vi "Lockin Engine.vi"(8 "error in (no error)":errorcluster, 9 "REF Waveforms":waveform(dbl)[](array[waveform]), 10 "AI Waveforms":waveform(dbl)[](array[waveform]), 11 "LockinDAQ":refnum<class "LockinDAQ.lvclass">) -> (0 "error out":errorcluster, 1 "SweepResults":T1, 2 "Averaged Results (X,Y,R,Theta,Mean)":T2 {"Results" format="%#_6p"}, 3 "LockinDAQ out":refnum<class "LockinDAQ.lvclass">)   [LabVIEW 2016, in "LockinDAQ.lvclass"]
uses:
  LockinDAQ.lvclass
  Typedefs/Results--Cluster.ctl
  Typedefs/SweepResults--Cluster.ctl
  LockinDAQ.lvclass/LockinDAQ.ctl
  <vilib>/Analysis/baseanly.llb/Mean (DBL).vi
  <vilib>/ptbypt/Filters.llb/Butterworth Filter PtByPt.vi
  <vilib>/Analysis/3filter.llb/Butterworth Filter.vi
  <vilib>/Analysis/3filter.llb/Butterworth Filter (DBL).vi
  <vilib>/addons/System Identification/Data Preprocess.llb/SI Lowpass Filter.vi
  <vilib>/addons/System Identification/Data Preprocess.llb/SI Lowpass Filter (SISO Waveform).vi
  <vilib>/addons/Digital Filter Design/Process.llb/DFD Filtering (Wfm NChan).vi
  <vilib>/measure/maresamp.llb/Resample Waveforms (single shot).vi
  <vilib>/measure/maresamp.llb/Resample Waveform (single shot).vi
  <vilib>/Analysis/NI_AALBase.lvlib
  <vilib>/addons/Digital Filter Design/NI_DigFilterLicensed.lvlib
panel:
  out "Results (Ch1)":cluster{i32[], dbl[]}[](graph)
  out "filter fC (Hz)":dbl=0.3183098861837907
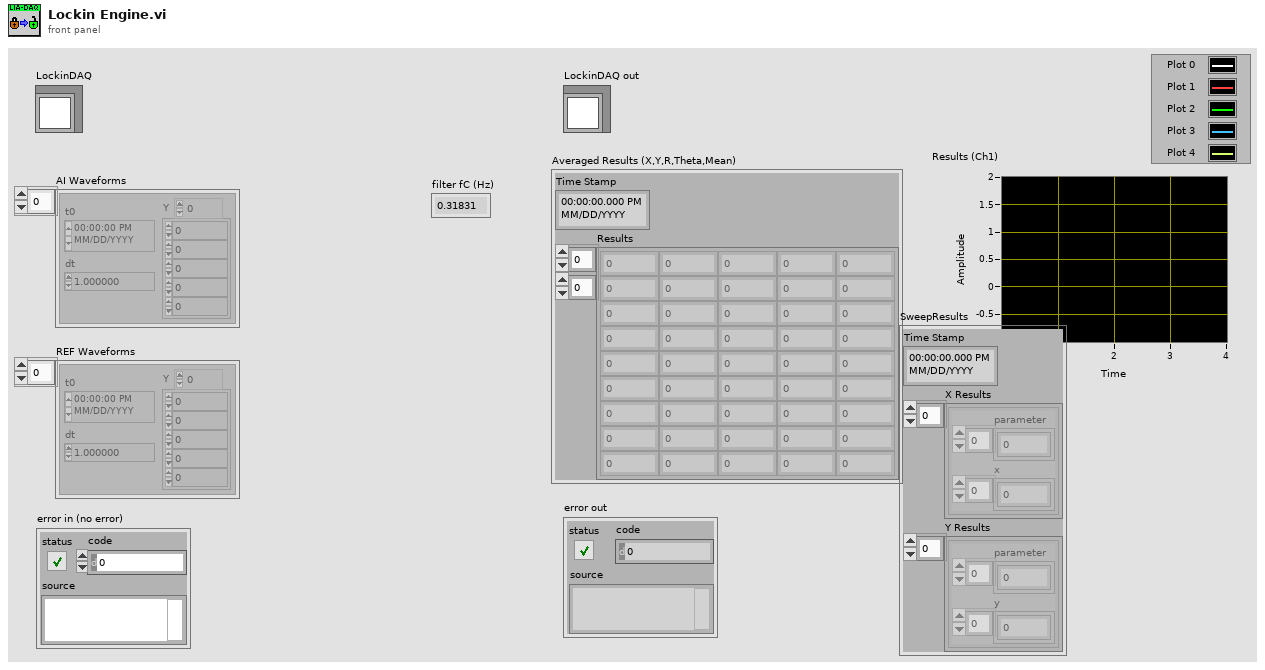
[diagram p1: front panel]
types:
  T1 = typedef "LockinDAQ.lvclass/SweepResults--Cluster.ctl" = cluster{"Time Stamp":timestamp, "X Results":cluster{"parameter":dbl[], "x":dbl[]}[], "Y Results":cluster{"parameter":dbl[], "y":dbl[]}[]}
  T2 = typedef "LockinDAQ.lvclass/Results--Cluster.ctl" = cluster{"Time Stamp":timestamp, "Results":dbl[][]}
  T3 = enum16{"method 1", "method 2", "method 3", "method 4", "method 5"}
  T4 = enum16{"Lowpass", "Highpass", "Bandpass", "Bandstop"}
  T5 = typedef "NI_DigFilterLicensed.lvlib/DFD Filter Obj.ctl" = cluster{"mSRate_Fs":dbl, "mSRate_Version":string, "mSRate_Comments":string, "mSRate_OrgCoef":T6, "mSRate_CurCoef":T6, "mSRate_Quantized?":bool, "mSRate_QCoef":T6, "mSRate_QSettings":T8[], "mSRate_Order":i32, "mSRate_Scaling":cluster{"mSRate_ScaleByPowerOf2?":bool, "mSRate_ScaleType":T10}}
  T6 = typedef "NI_DigFilterLicensed.lvlib/DFD Filter Coef.ctl" = cluster{"type":T7, "gain":dbl, "coef a (k)":dbl[], "coef b (v)":dbl[]}
  T7 = typedef "NI_DigFilterLicensed.lvlib/DFD Filter Structure Type Selector.ctl" = enum16{"Undefined", "FIR Direct Form", "FIR Direct Form Transposed", "FIR Symmetric", "FIR Antisymmetric", "IIR Direct Form I", "IIR Direct Form I Transposed", "IIR Direct Form II", "IIR Direct Form II Transposed", "IIR Cascaded Second Order Sections Form I", "IIR Cascaded Second Order Sections Form I Transposed", "IIR Cascaded Second Order Sections Form II", "IIR Cascaded Second Order Sections Form II Transposed", "Lattice Allpass (basic sections)", "Lattice Allpass (one multiplier sections)", "Lattice Allpass (normalized sections)", "Lattice AR (basic sections)", "Lattice AR (one multiplier sections)", "Lattice AR (normalized sections)", "Lattice MA (minimum phase)", "Lattice MA (maximum phase)", "Lattice ARMA (basic sections)", "Lattice ARMA (one multiplier sections)", "Lattice ARMA (normalized sections)"}
  T8 = typedef "NI_DigFilterLicensed.lvlib/dfd_Internal Quantization Settings.ctl" = cluster{"source":T9, "wl":i16, "iwl":i16, "overflow mode":enum16{"Saturation", "Wrap"}, "rounding mode":enum16{"Nearest", "Truncation"}, "signed?":bool}
  T9 = typedef "NI_DigFilterLicensed.lvlib/dfd_Internal Quantization Srcs.ctl" = u16
  T10 = typedef "NI_DigFilterLicensed.lvlib/DFD Coef Norm Type.ctl" = enum16{"No Norm", "Time Domain 1-Norm", "Time Domain 2-Norm", "Time Domain Inf-Norm"}
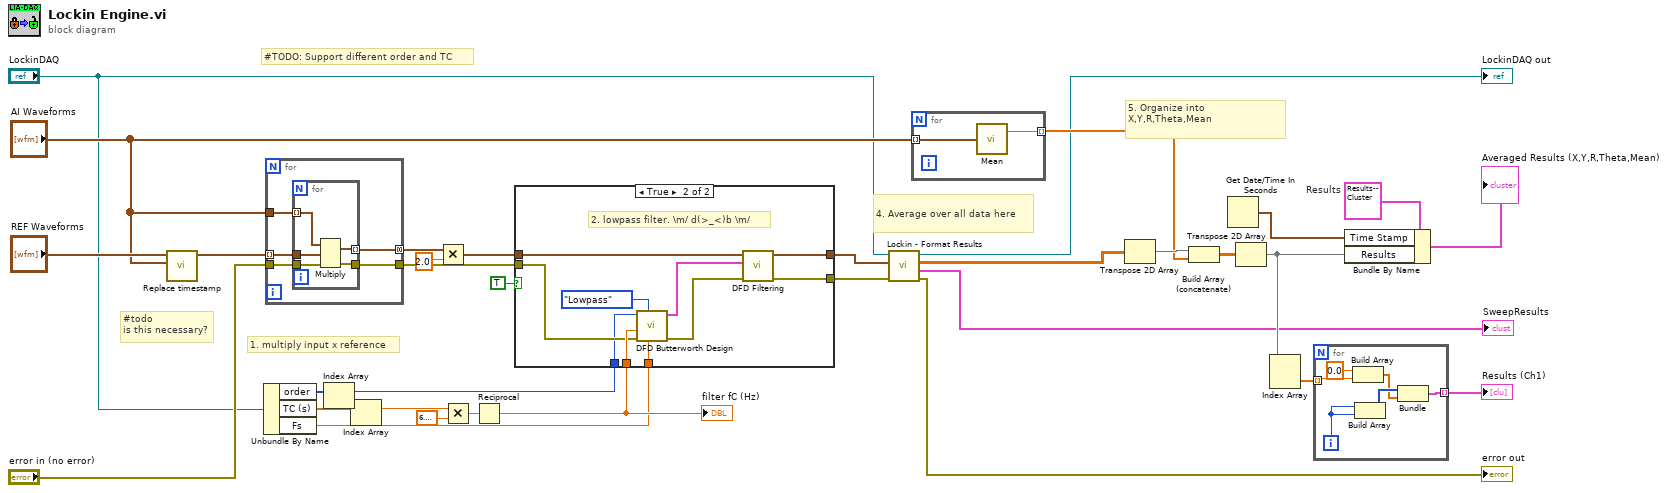
[diagram p0: block diagram]
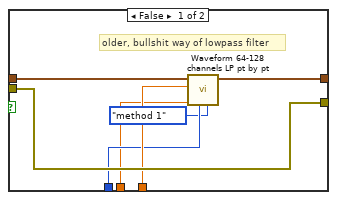
[diagram p2: hidden frame]
diagram:
  w27 = T2 {"Time Stamp"=timestamp(0 s since 1904-01-01), "Results"=[]}  # Results
  # "#TODO: Support different order and TC"
  # "#todo\nis this necessary?"
  # "5. Organize into X,Y,R,Theta,Mean"
  # "4. Average over all data here"
  # "1. multiply input x reference"
  n1 = call "Replace timestamp.vi"("Array in (use this time stamp)"="AI Waveforms", "Array in"="REF Waveforms") -> ("Array out"=w33:waveform(dbl)[])  [unwired: 9 in]
  n2 = Unbundle By Name("LockinDAQ") -> ("order"=w15:i32[], "TC (s)"=w30:dbl[], "Fs"=w16:dbl)
  n3 = for {
    tunnel: [w38] -> w24 mode=concatenating
    tunnel: w33 -> [w37] mode=indexing
    tunnel: "AI Waveforms" -> [w36]
    tunnel: [w35] -> w17
    tunnel: "error in (no error)" -> [w34]
    n4 = for {
      tunnel: w36 -> [w42] mode=indexing
      tunnel: w37 -> [w41]
      tunnel: [w43] -> w38 mode=indexing
      tunnel: [w40] -> w35
      tunnel: w34 -> [w39]
      n5 = Multiply(1:w41, 2:w42, 4:w39) -> (0:w43:waveform(dbl), 3:w40:errorcluster)
    }
  }
  n6 = Index Array(array=w15) -> (element=w2:i32)  [unwired: 1 in]
  n7 = Index Array(array=w30) -> (element=w1:dbl)  [unwired: 1 in]
  n8 = Multiply(x=w24, y=2.0) -> (x*y=w19:waveform(dbl)[])
  n9 = Multiply(x=w1, y=6.283185307179586) -> (x*y=w32:dbl)
  n10 = Reciprocal(x=w32) -> (1/x=w18:dbl)
  "filter fC (Hz)" <- w18
  n11 = case shown="True" TRUE {
    tunnel: w19 -> [w50 w58]
    tunnel: [w49 w57] -> w6
    tunnel: w18 -> [w45 w56]
    tunnel: w17 -> [w48 w55]
    tunnel: w16 -> [w47 w54]
    tunnel: w2 -> [w46 w53]
    tunnel: [w48 w51] -> w9
    frame False {
      # "older, bullshit way of lowpass filter"
      n12 = call "Waveform 64-128 channels LP pt by pt.vi"("Enum"=T3."method 1", "order"=w46, "fl"=w45, "fs"=w47, "Array in"=w50) -> ("Array out"=w49:waveform(dbl)[])  [unwired: 6 in]
    }
    frame True {
      # "2. lowpass filter. \\m/ d(>_<)b \\m/"
      n13 = call <vilib>:"DFD Butterworth Design.vi"("fs [Hz]"=w54, "filter type"=T4."Lowpass", "error in (no error)"=w55, "low cutoff freq [Hz]"=w56, "order"=w53) -> ("error out"=w59:errorcluster, "filter out"=w60:T5)  [unwired: 5 in]
      n14 = call-poly <vilib>:"DFD Filtering.vi"("error in (no error)"=w59, "filter"=w60, "signal in"=w58) -> ("error out"=w51:errorcluster, "signal out"=w57:waveform(dbl)[])  [unwired: 7 in]
    }
  }
  n15 = call "Lockin - Format Results.vi"("error in (no error)"=w9, "signal in"=w6, "LockinDAQ"="LockinDAQ") -> ("error out"=→"error out":errorcluster, "SweepResults"=→"SweepResults":T1, "Results (X,Y,R,Theta)"=w3:dbl[][], "LockinDAQ out"=→"LockinDAQ out":refnum<class "LockinDAQ.lvclass">)  [unwired: 5 in]
  n16 = for {
    tunnel: "AI Waveforms" -> [w62] mode=indexing
    tunnel: [w61] -> w28 mode=indexing
    n17 = call-poly <vilib>:"Mean.vi"("X"=w62) -> ("mean"=w61:dbl)  [unwired: 1 out]
  }
  n18 = Transpose 2D Array(2D array=w3) -> (transposed array=w29:dbl[][])
  n19 = Build Array (concatenate)(w29, w28) -> (w23:dbl[][])
  n20 = Get Date/Time In Seconds() -> (seconds since 1Jan1904=w26:timestamp)
  n21 = Transpose 2D Array(2D array=w23) -> (transposed array=w21:dbl[][])
  n22 = Index Array(array=w21) -> (element=w22:dbl[])  [unwired: 2 in]
  n23 = for {
    tunnel: w22 -> [w67] mode=indexing
    tunnel: [w63] -> w20 mode=indexing
    i -> [w68]
    n24 = Build Array(0.0 ("element"), w67) -> (w64:dbl[])
    n25 = Build Array(w68, w68) -> (w65:i32[])
    n26 = Bundle(w65, w64) -> (w63:cluster{i32[], dbl[]})  [unwired: 1 in]
  }
  "Results (Ch1)" <- w20
  n27 = Bundle By Name(cluster=w27, "Time Stamp"=w26, "Results"=w21) -> (→"Averaged Results (X,Y,R,Theta,Mean)":T2)
